vi "PrepareShootTactic_Init.vi"(0 "object in":refnum<class "PrepareShootTactic.lvclass">, 5 "error in (no error)":errorcluster) -> (14 "object out":refnum<class "PrepareShootTactic.lvclass">, 19 "error out":errorcluster)   [LabVIEW 2023, in "PrepareShootTactic.lvclass"]
uses:
  PrepareShootTactic.lvclass
  C:/Users/ebert/Documents/codes/SSL/repo/SSL_AI/KickTactic_class/KickTactic.lvclass
  C:/Users/ebert/Documents/codes/SSL/repo/SSL_AI/NewSTP/NewTactics/Tactic_v2_class/Tactic_v2.lvclass
  KickTactic_class/KickTactic_states_class/KickTactic_states.ctl
  NewSTP/NewSkills/HaltSkill_v2_class/HaltSkill_v2.lvclass
  C:/Users/ebert/Documents/codes/SSL/repo/SSL_AI/NewSTP/NewSkills/Skill_v2_class/Skill_v2.lvclass
  NewSTP/NewSkills/Skill_v2_class/Skill_v2.lvclass
  KickTactic_class/KickTactic.lvclass
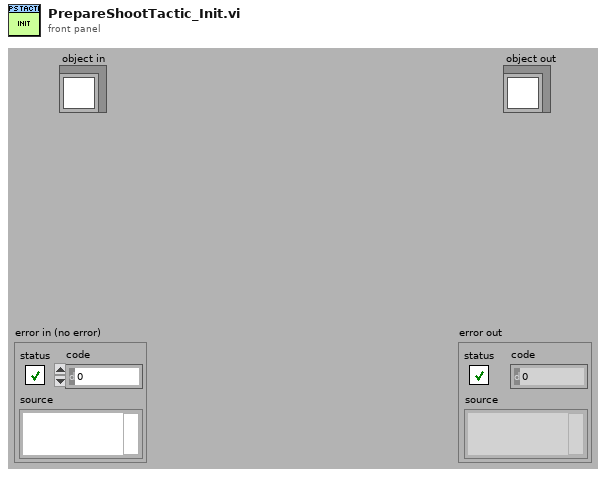
[diagram p1: front panel]
types:
  T1 = typedef "KickTactic.lvclass/KickTactic_states.ctl" = enum16{"GoToTangentPoint", "Circulate", "Align", "Kick"}
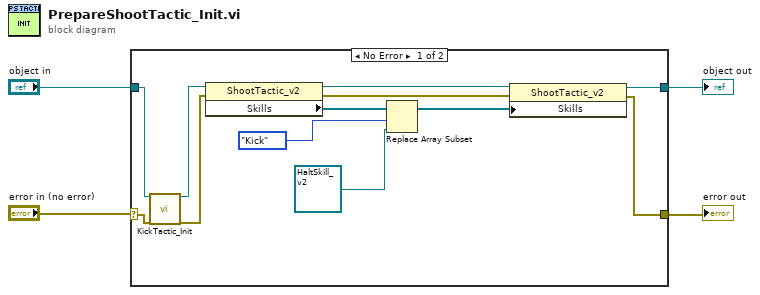
[diagram p0: block diagram]
diagram:
  n1 = case shown="No Error" "error in (no error)" {
    selector: "error in (no error)" -> [w8 w17]
    tunnel: "object in" -> [w16 w18]
    tunnel: [w10 w18] -> w3
    tunnel: [w5 w17] -> w1
    frame No Error {
      n2 = call "KickTactic_Init.vi"("object in"=w16, "error in (no error)"=w8) -> ("object out"=w11:refnum<class "PrepareShootTactic.lvclass">, "error out"=w7:errorcluster)  [unwired: 16 in]
      n3 = property class="ShootTactic_v2"(reference=w11, error in=w7) -> (reference out=w15:refnum<class "PrepareShootTactic.lvclass">, error out=w6:errorcluster, "Skills"=w14:refnum<class "Skill_v2.lvclass">[])
      n4 = Replace Array Subset(array=w14, new element=refnum<class "HaltSkill_v2.lvclass"> refnum ("HaltSkill_v2"), index=KickTactic_states."Kick" ("Enum")) -> (w12:refnum<class "Skill_v2.lvclass">[])
      n5 = property class="ShootTactic_v2"(reference=w15, error in=w6, "Skills"=w12) -> (reference out=w10:refnum<class "PrepareShootTactic.lvclass">, error out=w5:errorcluster)
    }
    frame Error {
    }
  }
  "object out" <- w3
  "error out" <- w1
